vi "Test Get Aggregated Code Coverage.vi"(8 "error in (no error)":errorcluster, 11 "Test Case In":refnum<class "Coverage Test.lvclass">) -> (0 "error out":errorcluster, 3 "Test Case Out":refnum<class "Coverage Test.lvclass">)   [LabVIEW 2020, in "LUnit Tests.lvlib" / "Coverage Test.lvclass"]
uses:
  Coverage Test.lvclass
  01074fa8-ee8a-411d-bc8b-fc92c4f90959.vi
  source/Framework/Coverage Analyzer/Coverage Analyzer.lvclass
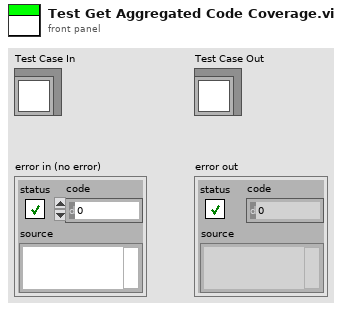
[diagram p1: front panel]
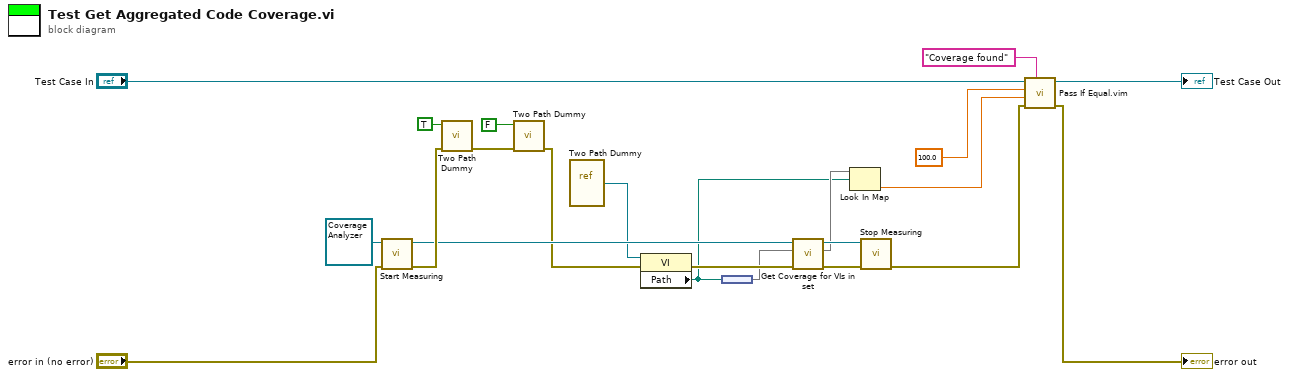
[diagram p0: block diagram]
diagram:
  n1 = call "Start Measuring.vi"("error in (no error)"="error in (no error)", "Coverage Analyzer in"=refnum<class "Coverage Analyzer.lvclass"> refnum) -> ("error out"=w14:errorcluster, "Coverage Analyzer out"=w9:refnum<class "Coverage Analyzer.lvclass">)  [unwired: 8 in]
  n2 = call "Two Path Dummy.vi"("error in (no error)"=w14, "Boolean"=TRUE) -> ("error out"=w18:errorcluster)  [unwired: 9 in]
  n3 = call "Two Path Dummy.vi"("error in (no error)"=w18, "Boolean"=FALSE) -> ("error out"=w6:errorcluster)  [unwired: 9 in]
  n4 = vi-ref "Two Path Dummy.vi"() -> (w4:refnum<vi>)
  n5 = property class="VI"(reference=w4, error in=w6) -> (error out=w5:errorcluster, "Path"=w2:path)  [unwired: 1 out]
  n6 = node(w2) -> (w1:set{path})
  n7 = call "Get Coverage for VIs in set.vi"("error in (no error)"=w5, "VIs"=w1, "Coverage Analyzer in"=w9) -> ("error out"=w10:errorcluster, "Code Coverage"=w7:map{path, dbl}, "Coverage Analyzer out"=w8:refnum<class "Coverage Analyzer.lvclass">)  [unwired: 6 in]
  n8 = Look In Map(map=w7, key=w2) -> (value=w3:dbl)  [unwired: 1 in, 1 out]
  n9 = call "Stop Measuring.vi"("error in (no error)"=w10, "Coverage Analyzer in"=w8) -> ("error out"=w12:errorcluster)  [unwired: 8 in, 1 out]
  n10 = call "Pass If Equal.vim"("Description"="Coverage found", "error in (no error)"=w12, "Actual"=w3, "Expected"=100.0 ("Coverage Percentage"), "LUnit Test Case In"="Test Case In") -> ("error out"=→"error out":errorcluster, "LUnit Test Case Out"=→"Test Case Out":refnum<class "Coverage Test.lvclass">)  [unwired: 5 in]
